vi "Trial v5.vi"(2 "error in (no error)":errorcluster, 3 "queue in":refnum<queue>, 4 "DDA":bool=TRUE) -> (0 "error out":errorcluster, 1 "queue out":refnum<queue>)   [LabVIEW 2017]
uses:
  Control/RPY.ctl
  <vilib>/Analysis/baseanly.llb/Real Dot Product.vi
  <vilib>/Analysis/_algsub.llb/Real Vector Norm.vi
  <vilib>/Analysis/baseanly.llb/Outer Product.vi
  <vilib>/Analysis/baseanly.llb/Real Outer Product.vi
  <vilib>/robotics/Kinematics/Create Lie Group Matrix.vi
  SubVI/Global.vi
  <vilib>/Analysis/7linalg.llb/Create Special Matrix.vi
  <vilib>/Analysis/7linalg.llb/Create Special Real Matrix.vi
  <vilib>/Analysis/Matrix/Numeric/Multiply/Multiply.vi
  <vilib>/Analysis/Matrix/Numeric/Multiply/Multiply - RM,R.vi
  <vilib>/Analysis/Matrix/Numeric/Multiply/Multiply - R,RM.vi
  <vilib>/Analysis/Matrix/Numeric/Add/Add.vi
  <vilib>/Analysis/Matrix/Numeric/Add/Add - RM,RM.vi
  <vilib>/Analysis/NI_AALPro.lvlib
  <vilib>/robotics/Kinematics/NI_Kinematics.lvlib
  Control/Damping.ctl
  <vilib>/Analysis/NI_AALBase.lvlib
  <vilib>/ptbypt/NI_PtbyPt.lvlib
panel:
  in  "gamma":dbl=0.1
  in  "k":i32=5
  in  "n":i32=1
  in  "alpha theta":dbl=0.1
  in  "alpha w":dbl=0.1
  in  "lambda theta":dbl=0.9
  in  "lambda w":dbl=0.9
  in  "alpha Rbar":dbl=0.1
  in  "RoM (deg)":dbl=75.0 format="%#_13g"
  in  "Variable":T1
  in  "Time":dbl=5.0 caption="Time Target (s)"
  in  "epsilon":dbl=0.1
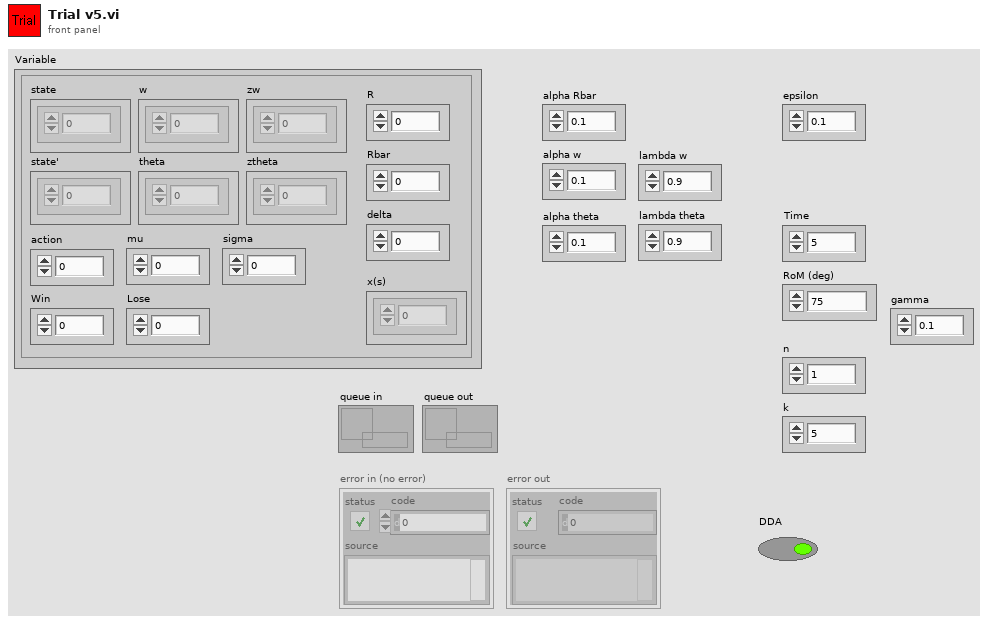
[diagram p1: front panel]
types:
  T1 = cluster{"w":dbl[], "theta":dbl[], "R":dbl, "Rbar":dbl, "zw":dbl[], "ztheta":dbl[], "action":dbl, "state":dbl[], "state'":dbl[], "delta":dbl, "mu":dbl, "sigma":dbl, "x(s)":dbl[], "Win":dbl, "Lose":dbl}
  T2 = typedef "RPY.ctl" = cluster{"roll":dbl, "pitch":dbl, "yaw":dbl}
  T3 = typedef "Damping.ctl" = cluster{"Cx":dbl, "Cy":dbl, "Cz":dbl}
  T4 = typedef "NI_Matrix.lvlib/RealMatrix.ctl" = dbl[][]
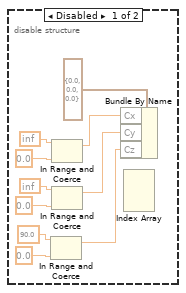
[diagram p2: hidden frame]
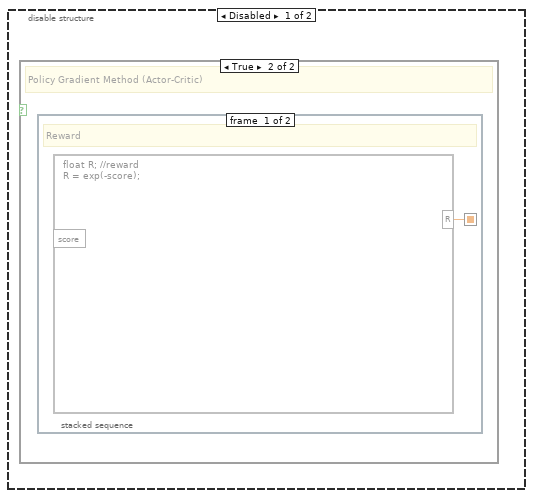
[diagram p3: hidden frame]
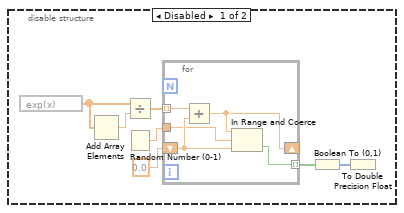
[diagram p6: hidden frame]
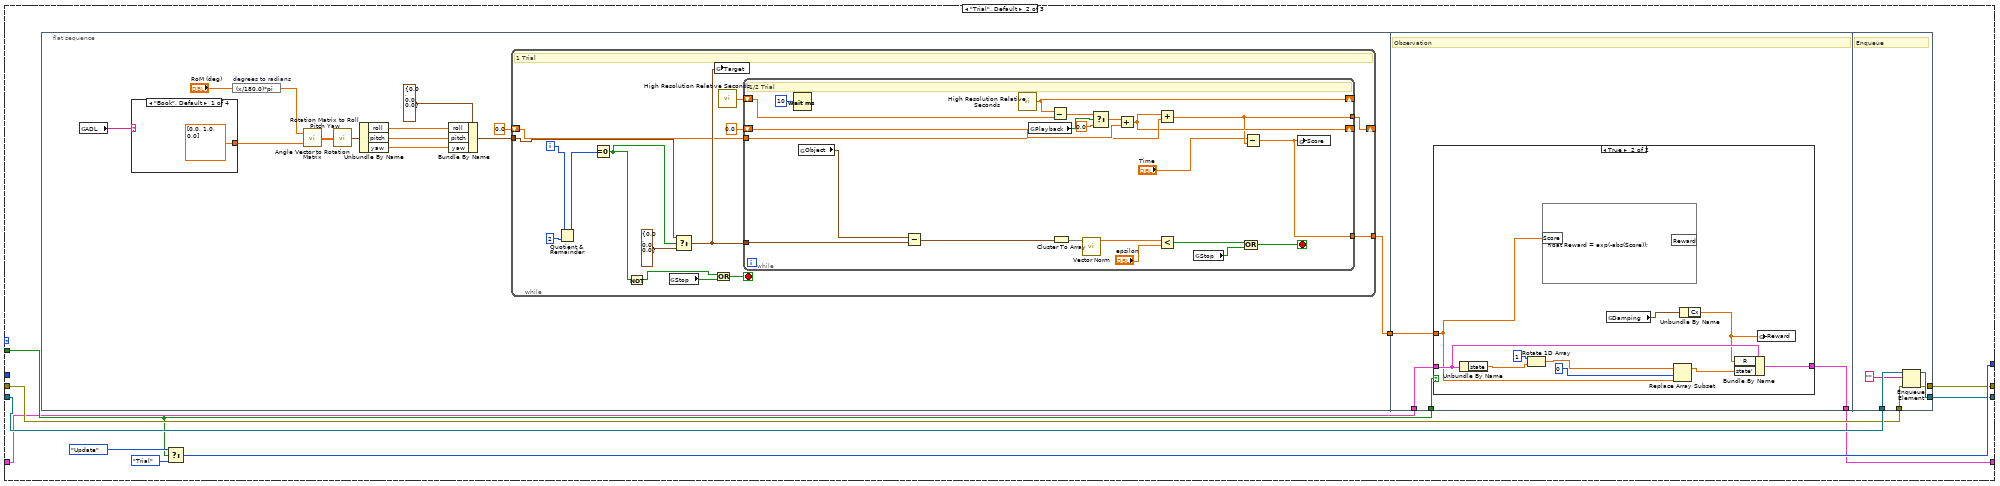
[diagram p7: hidden frame]
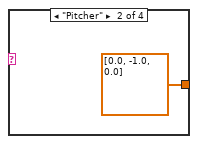
[diagram p8: hidden frame]
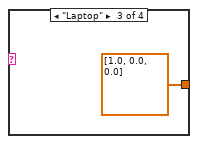
[diagram p9: hidden frame]
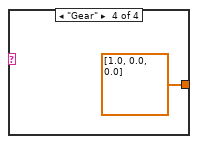
[diagram p10: hidden frame]
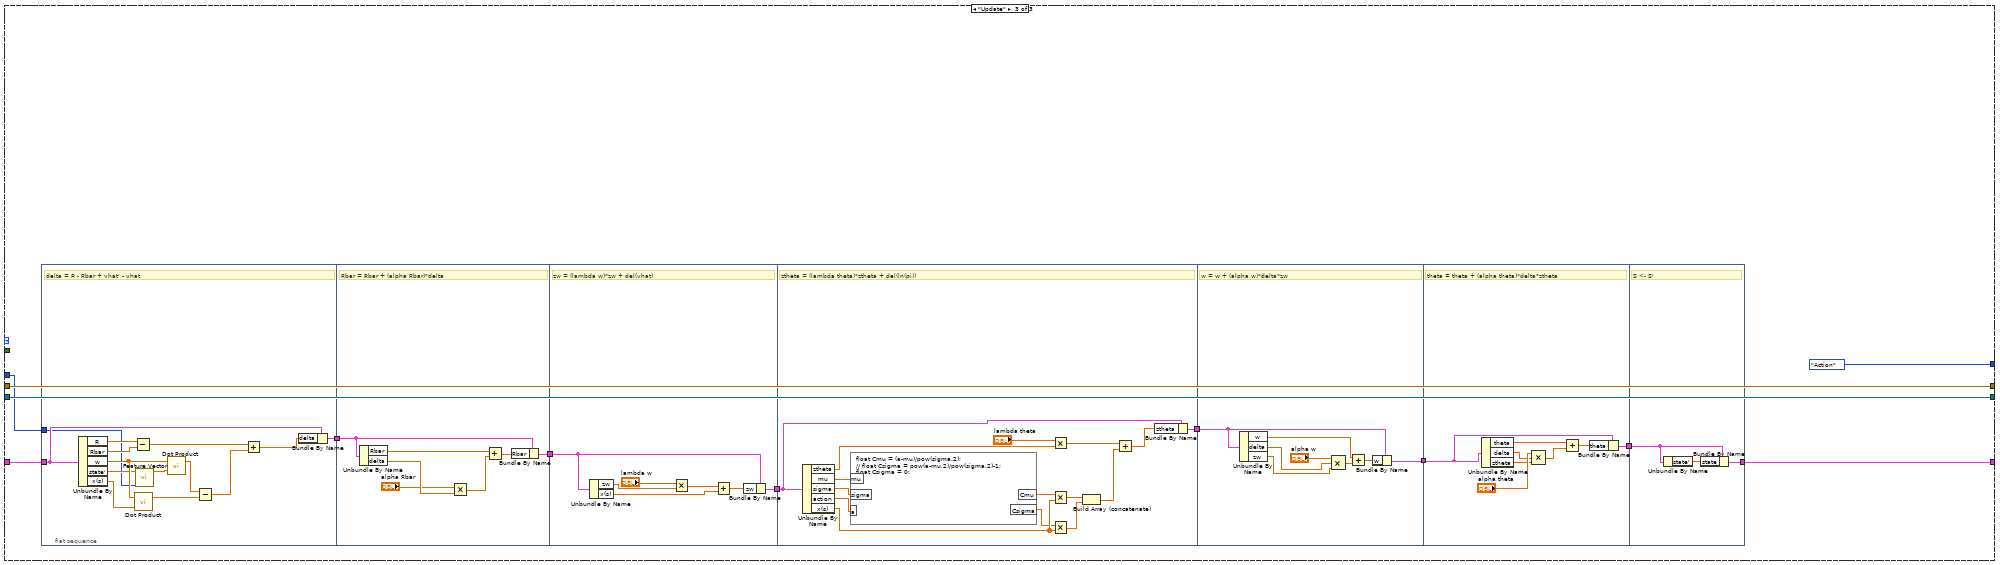
[diagram p12: hidden frame]
diagram:
  n1 = flat-sequence {
    tunnel: "error in (no error)" -> [w13]
    tunnel: "queue in" -> [w15]
    tunnel: "DDA" -> [w8]
    tunnel: [w14] -> w2
    tunnel: [w12] -> w1
    frame #0 {
      n2 = flat-sequence {
        tunnel: [w27] -> w7
        tunnel: ["n"] -> w6
        frame #0 {
          n3 = Initialize Array(2.220446049250313e-16, "k") -> (w18:dbl[])
          n4 = call "Feature Vector.vi"("n"="n", "state"=w18) -> ("x(s)"=w24:dbl[])  [unwired: 9 in]
          n5 = Array Size(array=w24) -> (size(s)=w23:i32)
          n6 = Initialize Array(0.0 ("element"), w23) -> (w21:dbl[])
          n7 = Build Array (concatenate)(w21, w21) -> (w25:dbl[])
          n8 = Bundle By Name(cluster="Variable", "w"=w21, "zw"=w21, "theta"=w25, "ztheta"=w25, "state"=w18, "Rbar"=0.0) -> (w27:T1)
        }
      }
      n9 = Select(t=enum16{"Action", "Trial", "Update"}."Action", s=w8, f=enum16{"Action", "Trial", "Update"}."Trial") -> (s? t:f=w9:enum16{"Action", "Trial", "Update"})
      n10 = while {
        shift-right: [w32] -> w14
        shift-left: w15 -> [w34]
        shift-right: [w31] -> w12
        shift-left: w13 -> [w33]
        shift-right: [w36] -> _
        shift-left: w9 -> [w37]
        tunnel: w8 -> [w35]
        shift-right: [w29] -> _
        shift-left: w7 -> [w30]
        tunnel: w6 -> [w28]
        stop <- w38 stop-if-true
        # "State Machine"
        n11 = case shown="\"Action\"" w37 {
          tunnel: [enum16{"Action", "Trial", "Update"}."Trial" w72 enum16{"Action", "Trial", "Update"}."Action"] -> w36
          tunnel: w35 -> [_ w66 _]
          tunnel: w34 -> [w53 w71 w157]
          tunnel: w33 -> [w54 w67 w158]
          tunnel: [w53 w70 w157] -> w32
          tunnel: [w54 w69 w158] -> w31
          tunnel: w30 -> [w45 w65 w156]
          tunnel: [w39 w64 w155] -> w29
          tunnel: w28 -> [w42 _ w148]
          frame "Action" {
            n12 = Unbundle By Name(w45) -> ("theta"=w52:dbl[], "state"=w46:dbl[])
            n13 = call "Feature Vector.vi"("n"=w42, "state"=w46) -> ("x(s)"=w43:dbl[])  [unwired: 9 in]
            n14 = Array Size(array=w43) -> (size(s)=w51:i32)
            n15 = Split 1D Array(array=w52, index=w51) -> (first subarray=w50:dbl[], second subarray=w49:dbl[])
            n16 = call-poly <vilib>:"Dot Product.vi"("Y Vector"=w43, "X Vector"=w50) -> ("X * Y"=w41:dbl)  [unwired: 1 out]
            n17 = call-poly <vilib>:"Dot Product.vi"("Y Vector"=w43, "X Vector"=w49) -> ("X * Y"=w48:dbl)  [unwired: 1 out]
            n18 = Exponential(1:w48) -> (0:w40:dbl)
            n19 = call <vilib>:"Gaussian White Noise PtByPt.vi"("standard deviation"=w40) -> ("Gaussian white noise"=w47:dbl)  [unwired: 2 in]
            n20 = Add(x=w41, y=w47) -> (x+y=w44:dbl)
            n21 = flat-sequence {
              tunnel: w44 -> [w59]
              frame #0 {
                # "Adjust Damping"
                n22 = Multiply(x="gamma", y=w59) -> (x*y=w57:dbl)
                n23 = global read "Global.vi" "Damping"() -> (w62:T3)
                n24 = Unbundle By Name(w62) -> ("Cx"=w60:dbl)
                n25 = Add(x=w57, y=w60) -> (x+y=w56:dbl)
                n26 = Bundle By Name(cluster=w62, "Cx"=w56) -> (w61:T3)
                n27 = global write "Global.vi" "Damping"(w61) -> ()
              }
            }
            n28 = Bundle By Name(cluster=w45, "mu"=w41, "sigma"=w40, "action"=w44, "x(s)"=w43) -> (w39:T1)
          }
          frame "Trial", Default {
            n29 = flat-sequence {
              tunnel: [w74] -> w63
              tunnel: w66 -> [w131]
              tunnel: w65 -> [w130]
              tunnel: [w129] -> w64
              tunnel: w63 -> [w128]
              tunnel: w71 -> [w147]
              tunnel: [w146] -> w70
              tunnel: [w145] -> w69
              tunnel: w67 -> [w143]
              frame #0 {
                n30 = global read "Global.vi" "ADL"() -> (w78:string)
                n31 = case shown="\"Book\", Default" w78 {
                  tunnel: [dbl[] [0.0, 1.0, 0.0] dbl[] [0.0, -1.0, 0.0] dbl[] [1.0, 0.0, 0.0] dbl[] [1.0, 0.0, 0.0]] -> w77
                  frame "Book", Default {
                  }
                  frame "Pitcher" {
                  }
                  frame "Laptop" {
                  }
                  frame "Gear" {
                  }
                }
                n32 = expression code="(x/180.0)*pi" "degrees to radians"("RoM (deg)") -> (w75:dbl)
                n33 = call <vilib>:"Angle Vector to Rotation Matrix.vi"("vector"=w77, "angle"=w75) -> ("rotation matrix"=w81:T4)
                n34 = call <vilib>:"Rotation Matrix to Roll Pitch Yaw.vi"("rotation matrix"=w81) -> ("angles"=w82:cluster{"roll":dbl, "pitch":dbl, "yaw":dbl})
                n35 = Unbundle By Name(w82) -> ("roll"=w83:dbl, "pitch"=w84:dbl, "yaw"=w85:dbl)
                n36 = Bundle By Name(cluster=T2 {"roll"=0.0, "pitch"=0.0, "yaw"=0.0} ("Target"), "roll"=w83, "pitch"=w84, "yaw"=w85) -> (w79:T2)
                n37 = while {
                  tunnel: w79 -> [w100]
                  shift-right: [w92] -> _
                  shift-left: 0.0 -> [w93]
                  tunnel: [w91] -> w74
                  i -> [w103]
                  stop <- w96 stop-if-true
                  # "1 Trial"
                  n38 = Quotient & Remainder(x=w103, y=2) -> (x-y*floor(x/y)=w101:i32)  [unwired: 1 out]
                  n39 = Equal To 0?(x=w101) -> (x = 0?=w95:bool)
                  n40 = Not(x=w95) -> (.not. x?=w94:bool)
                  n41 = global read "Global.vi" "Stop"() -> (w97:bool)
                  n42 = Select(t=w100, s=w95, f=T2 {"roll"=0.0, "pitch"=0.0, "yaw"=0.0} ("Target")) -> (s? t:f=w98:T2)
                  n43 = global write "Global.vi" "Target"(w98) -> ()
                  n44 = Or(x=w94, y=w97) -> (x .or. y?=w96:bool)
                  n45 = call <vilib>:"High Resolution Relative Seconds.vi"() -> ("relative seconds"=w105:dbl)
                  n46 = while {
                    tunnel: w98 -> [w115]
                    shift-right: [w121] -> _
                    shift-left: w105 -> [w122]
                    shift-right: [w113] -> _
                    shift-left: 0.0 -> [w120]
                    tunnel: w93 -> [w114]
                    tunnel: [w111] -> w92
                    tunnel: [w107] -> w91
                    stop <- w108 stop-if-true
                    # "1/2 Trial"
                    n47 = Wait (ms)(milliseconds to wait=u32 10) -> ()  [unwired: 1 out]
                    n48 = global read "Global.vi" "Object"() -> (w125:T2)
                    n49 = Subtract(x=w125, y=w115) -> (x-y=w126:T2)
                    n50 = call <vilib>:"High Resolution Relative Seconds.vi"() -> ("relative seconds"=w121:dbl)
                    n51 = global read "Global.vi" "Playback"() -> (w119:bool)
                    n52 = Subtract(x=w121, y=w122) -> (x-y=w118:dbl)
                    n53 = Cluster To Array(cluster=w126) -> (array=w127:dbl[])
                    n54 = call-poly <vilib>:"Vector Norm.vi"("Input Vector"=w127) -> ("norm"=w124:dbl)  [unwired: 9 in, 1 out]
                    n55 = Select(t=w118, s=w119, f=0.0) -> (s? t:f=w117:dbl)
                    n56 = Add(x=w117, y=w120) -> (x+y=w113:dbl)
                    n57 = Add(x=w113, y=w114) -> (x+y=w111:dbl)
                    n58 = Less?(x=w124, y="epsilon") -> (x < y?=w110:bool)
                    n59 = global read "Global.vi" "Stop"() -> (w109:bool)
                    n60 = Subtract(x="Time", y=w111) -> (x-y=w107:dbl)
                    n61 = Compound Arithmetic op=OR(w110, w109) -> (w108:bool)
                    n62 = global write "Global.vi" "Score"(w107) -> ()
                  }
                }
              }
              frame #1 {
                # "Observation"
                n63 = case shown="True" w131 {
                  tunnel: w130 -> [w132 w141]
                  tunnel: [w132 w142] -> w129
                  tunnel: w128 -> [_ w135]
                  frame False {
                  }
                  frame True {
                    n64 = Unbundle By Name(w141) -> ("state"=w139:dbl[])
                    n65 = Rotate 1D Array(1:w139, 2:1 ("n")) -> (0:w138:dbl[])
                    n66 = formula code="float Reward = exp(-abs(Score));"("Score"=w135) -> ()  [unwired: 1 out]
                    n67 = global read "Global.vi" "Damping"() -> (w134:T3)
                    n68 = Replace Array Subset(array=w138, new element=w135, index=0) -> (w136:dbl[])
                    n69 = Unbundle By Name(w134) -> ("Cx"=w133:dbl)
                    n70 = Bundle By Name(cluster=w141, "R"=w133, "state'"=w136) -> (w142:T1)
                    n71 = global write "Global.vi" "Reward"(w133) -> ()
                  }
                }
              }
              frame #2 {
                # "Enqueue"
                n72 = Enqueue Element(queue=w147, element="", error in (no error)=w143) -> (queue out=w146:refnum<queue>, error out=w145:errorcluster)  [unwired: 1 in, 1 out]
              }
            }
            n73 = Select(t=enum16{"Action", "Trial", "Update"}."Update", s=w66, f=enum16{"Action", "Trial", "Update"}."Trial") -> (s? t:f=w72:enum16{"Action", "Trial", "Update"})
          }
          frame "Update" {
            n74 = flat-sequence {
              tunnel: [w163] -> w154
              tunnel: w156 -> [w165]
              tunnel: w148 -> [w160]
              tunnel: w154 -> [w176]
              tunnel: [w174] -> w153
              tunnel: w153 -> [w184]
              tunnel: [w182] -> w152
              tunnel: w152 -> [w190]
              tunnel: [w188] -> w151
              tunnel: w151 -> [w205]
              tunnel: [w203] -> w150
              tunnel: w150 -> [w212]
              tunnel: [w211] -> w149
              tunnel: [w219] -> w155
              tunnel: w149 -> [w221]
              frame #0 {
                # "delta = R - Rbar + vhat' - vhat"
                n75 = Unbundle By Name(w165) -> ("R"=w173:dbl, "Rbar"=w172:dbl, "w"=w170:dbl[], "state'"=w162:dbl[], "x(s)"=w161:dbl[])
                n76 = Subtract(x=w173, y=w172) -> (x-y=w167:dbl)
                n77 = call-poly <vilib>:"Dot Product.vi"("Y Vector"=w161, "X Vector"=w170) -> ("X * Y"=w168:dbl)  [unwired: 1 out]
                n78 = call "Feature Vector.vi"("n"=w160, "state"=w162) -> ("x(s)"=w171:dbl[])  [unwired: 9 in]
                n79 = call-poly <vilib>:"Dot Product.vi"("Y Vector"=w171, "X Vector"=w170) -> ("X * Y"=w169:dbl)  [unwired: 1 out]
                n80 = Subtract(x=w169, y=w168) -> (x-y=w166:dbl)
                n81 = Add(x=w167, y=w166) -> (x+y=w164:dbl)
                n82 = Bundle By Name(cluster=w165, "delta"=w164) -> (w163:T1)
              }
              frame #1 {
                # "Rbar = Rbar + (alpha Rbar)*delta"
                n83 = Unbundle By Name(w176) -> ("Rbar"=w180:dbl, "delta"=w179:dbl)
                n84 = Multiply(x="alpha Rbar", y=w179) -> (x*y=w178:dbl)
                n85 = Add(x=w180, y=w178) -> (x+y=w175:dbl)
                n86 = Bundle By Name(cluster=w176, "Rbar"=w175) -> (w174:T1)
              }
              frame #2 {
                # "zw = (lambda w)*zw + del(vhat)"
                n87 = Unbundle By Name(w184) -> ("zw"=w187:dbl[], "x(s)"=w181:dbl[])
                n88 = Multiply(x="lambda w", y=w187) -> (x*y=w185:dbl[])
                n89 = Add(x=w185, y=w181) -> (x+y=w183:dbl[])
                n90 = Bundle By Name(cluster=w184, "zw"=w183) -> (w182:T1)
              }
              frame #3 {
                # "ztheta = (lambda theta)*ztheta + del(ln(pi))"
                n91 = Unbundle By Name(w190) -> ("ztheta"=w202:dbl[], "mu"=w200:dbl, "sigma"=w199:dbl, "action"=w198:dbl, "x(s)"=w196:dbl[])
                n92 = formula code="float Cmu = (a-mu)/pow(sigma,2);\n// float Csigma = pow(a-mu,2)/pow(sigma,2)-1;\nfloat Csigma = 0;"("mu"=w200, "sigma"=w199, "a"=w198) -> ("Cmu"=w197:dbl, "Csigma"=w195:dbl)
                n93 = Multiply(x="lambda theta", y=w202) -> (x*y=w192:dbl[])
                n94 = Multiply(x=w197, y=w196) -> (x*y=w194:dbl[])
                n95 = Multiply(x=w195, y=w196) -> (x*y=w193:dbl[])
                n96 = Build Array (concatenate)(w194, w193) -> (w191:dbl[])
                n97 = Add(x=w192, y=w191) -> (x+y=w189:dbl[])
                n98 = Bundle By Name(cluster=w190, "ztheta"=w189) -> (w188:T1)
              }
              frame #4 {
                # "w = w + (alpha w)*delta*zw"
                n99 = Unbundle By Name(w205) -> ("w"=w210:dbl[], "delta"=w209:dbl, "zw"=w208:dbl[])
                n100 = Compound Arithmetic op=MULTIPLY("alpha w", w209, w208) -> (w206:dbl[])
                n101 = Add(x=w210, y=w206) -> (x+y=w204:dbl[])
                n102 = Bundle By Name(cluster=w205, "w"=w204) -> (w203:T1)
              }
              frame #5 {
                # "theta = theta + (alpha theta)*delta*ztheta"
                n103 = Unbundle By Name(w212) -> ("theta"=w213:dbl[], "delta"=w214:dbl, "ztheta"=w215:dbl[])
                n104 = Compound Arithmetic op=MULTIPLY("alpha theta", w214, w215) -> (w217:dbl[])
                n105 = Add(x=w213, y=w217) -> (x+y=w218:dbl[])
                n106 = Bundle By Name(cluster=w212, "theta"=w218) -> (w211:T1)
              }
              frame #6 {
                # "S <- S'"
                n107 = Unbundle By Name(w221) -> ("state'"=w220:dbl[])
                n108 = Bundle By Name(cluster=w221, "state"=w220) -> (w219:T1)
              }
            }
          }
        }
        n109 = global read "Global.vi" "Stop"() -> (w38:bool)
      }
    }
  }
  n110 = disable-structure shown="Enabled" {
    frame Disabled {
      n111 = In Range and Coerce(upper limit=90.0, lower limit=0.0) -> (coerced(x)=w231:dbl)  [unwired: 1 in, 1 out]
      n112 = In Range and Coerce(upper limit=inf, lower limit=0.0) -> (coerced(x)=w229:dbl)  [unwired: 1 in, 1 out]
      n113 = In Range and Coerce(upper limit=inf, lower limit=0.0) -> (coerced(x)=w230:dbl)  [unwired: 1 in, 1 out]
      n114 = Bundle By Name(cluster=T3 {"Cx"=0.0, "Cy"=0.0, "Cz"=0.0} ("State"), "Cx"=w229, "Cy"=w230, "Cz"=w231) -> ()  [unwired: 1 out]
      n115 = Index Array() -> ()  [unwired: 4 in, 3 out]
    }
    frame Enabled {
    }
  }
  n116 = disable-structure shown="Enabled" {
    frame Disabled {
      n117 = expression code="exp(x)"() -> (w234:dbl[])  [unwired: 1 in]
      n118 = Add Array Elements(numeric array=w234) -> (sum=w235:dbl)
      n119 = Divide(x=w234, y=w235) -> (x/y=w232:dbl[])
      n120 = Random Number (0-1)() -> (number: 0 to 1=w236:dbl)
      n121 = for {
        shift-right: [w242] -> _
        shift-left: 0.0 -> [w243]
        tunnel: w236 -> [w241]
        tunnel: [w240] -> w237 mode=indexing
        tunnel: w232 -> [w239] mode=indexing
        n122 = Add(x=w239, y=w243) -> (x+y=w242:dbl)
        n123 = In Range and Coerce(upper limit=w242, x=w241, lower limit=w243) -> (In Range?=w240:bool)  [unwired: 1 out]
      }
      n124 = Boolean To (0,1)(Boolean=w237) -> (0, 1=w238:i16[])
      n125 = To Double Precision Float(number=w238) -> ()  [unwired: 1 out]
    }
    frame Enabled {
    }
  }
  n126 = disable-structure shown="Enabled" {
    frame Disabled {
      n127 = case shown="True" {
        selector: _ -> [_ _]
        frame False {
        }
        frame True {
          # "Policy Gradient Method (Actor-Critic)"
          n128 = stacked-sequence {
            seq-local: [w244 _] -> [_ _]
            frame #0 {
              # "Reward"
              n129 = formula code="float R; //reward\nR = exp(-score);"() -> ("R"=w244:dbl)  [unwired: 1 in]
            }
            frame #1 {
            }
          }
        }
      }
    }
    frame Enabled {
    }
  }
  "error out" <- w1
  "queue out" <- w2
